vi "AOTF-Trigger_1.vi"(0 "Channel":string="1", 1 "Pulse length":i16[](array[numeric]), 2 "Sync trigger ratio":i32=20, 3 "error in (no error)":errorcluster caption="Fehler (Eingang, kein Fehler)", 4 "Triggered":bool, 5 "lp":dbl, 6 "ap":dbl) -> (7 "error out":errorcluster caption="Fehler (Ausgang)")   [LabVIEW 2011]
doc: "I. Description:\nThis example demonstrates how to generate a continuous digital pulse train from a Counter Output Channel started by an external digital trigger. The Frequency, Duty Cycle, and Idle State are all configurable. \n\nThis example shows how to configure the pulse in terms of Frequency/Duty Cycle, but can easily be modified to generate a pulse in terms of Time or Ticks.\n\nII. Instructions for Running:\n1. Select the Physical Channel which corresponds to the counter you want to output your signal to on the DAQ device.\n2. Enter the Frequency and Duty Cycle to define the pulse parameters. You can also change the Idle State to set the state the line will remain in after the generation is stopped. Additionally, you can set the Initial Delay (in seconds) which will delay the beginning of the pulse train from the start call; this is currently wired to 0.0 on the block diagram. \n3. Setup the Trigger Parameters. In this example the VI is expecting a Rising Edge Digital Trigger on PFI9. \n\nIII. Block Diagram Steps:\n1. Create a Counter Output channel to produce a Pulse in terms of Frequency. If the Idle State of the pulse is set to low the first transition of the generated signal is from low to high.\n2. Use the DAQmx Trigger VI to configure a trigger to start on a digital edge.\n2. Use the DAQmx Timing VI (Implicit) to configure the duration of the pulse generation.\n3. Call the Start VI to arm the counter and begin the pulse train generation.\n4. Loop continuously until the user presses the Stop button. Check for errors every 100 ms using the Is Task Done? VI\n5. Call the Clear Task VI to clear the Task.\n\nIV. I/O Connections Overview:\nThe counter will output the pulse train on the output terminal of the counter specified in the Physical Channel I/O control. \n\nIn this example the output will be sent to the default output terminal on ctr0.\n\nFor more information on the default counter input and output terminals for your device, open the NI-DAQmx Help, and refer to Counter Signal Connections found under the Device Considerations book in the table of contents."
uses:
  <vilib>/DAQmx/configure/timing.llb/DAQmx Timing (Implicit).vi
  <vilib>/Utility/error.llb/DialogType.ctl
  <vilib>/DAQmx/configure/trigger.llb/DAQmx Start Trigger (Digital Edge).vi
  <vilib>/DAQmx/write.llb/DAQmx Write (Digital Bool 1Line 1Point).vi
  <vilib>/DAQmx/read.llb/DAQmx Read (Digital Bool 1Line 1Point).vi
  <vilib>/DAQmx/create/channels.llb/DAQmx Create Channel (DI-Digital Input).vi
  <vilib>/DAQmx/create/channels.llb/DAQmx Create Channel (DO-Digital Output).vi
  <vilib>/DAQmx/create/channels.llb/DAQmx Create Channel (CO-Pulse Generation-Ticks).vi
  <vilib>/DAQmx/create/channels.llb/DAQmx Create Channel (CO-Pulse Generation-Frequency).vi
  <vilib>/DAQmx/create/channels.llb/DAQmx Create Channel (CO-Pulse Generation-Time).vi
panel:
  out "Delay":dbl[](array[numeric])
  out "Duty cycle":dbl[](array[numeric])
  # "Channel Parameters"
  # "Trigger Parameters"
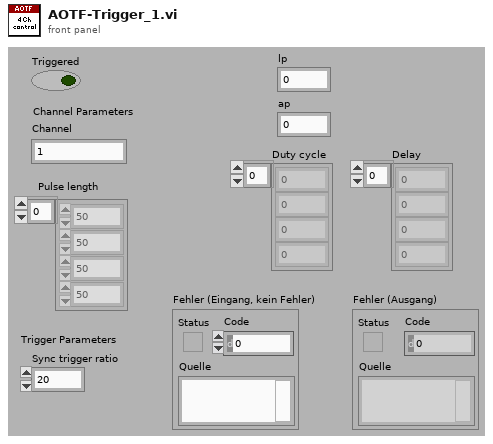
[diagram p1: front panel]
types:
  T1 = typedef "DialogType.ctl" = u16
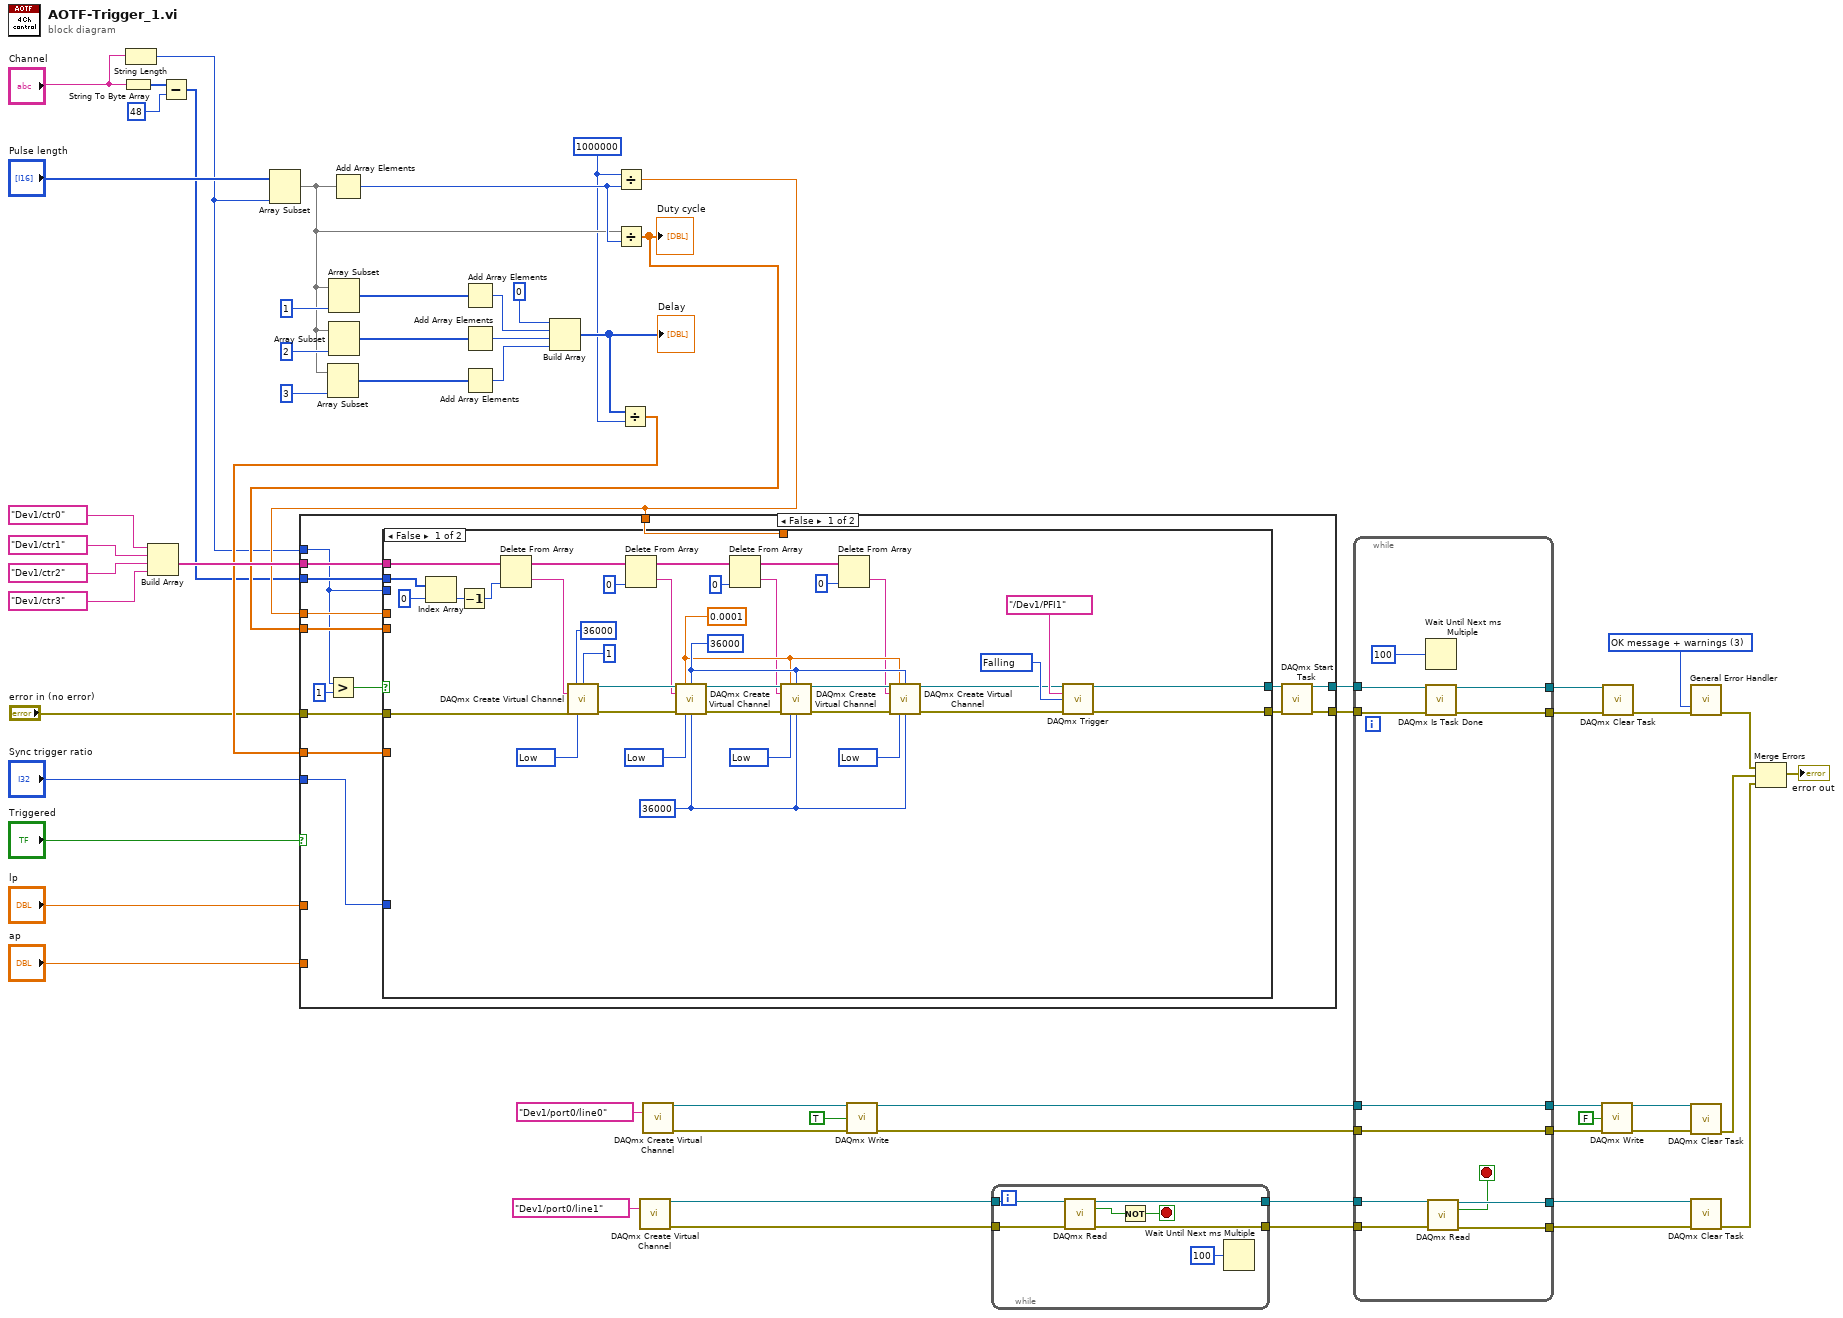
[diagram p0: block diagram]
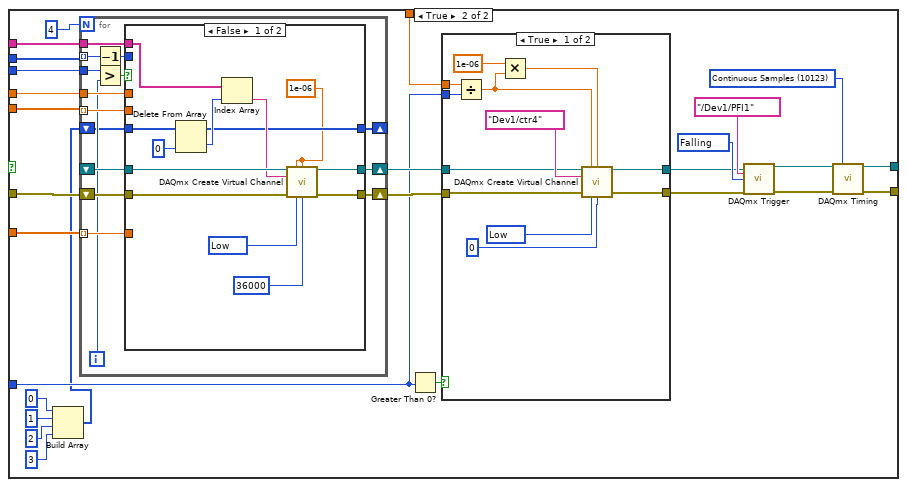
[diagram p2: hidden frame]
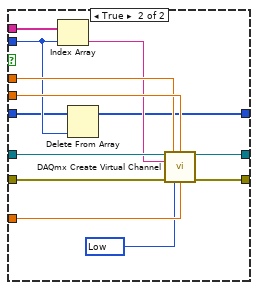
[diagram p4: hidden frame]
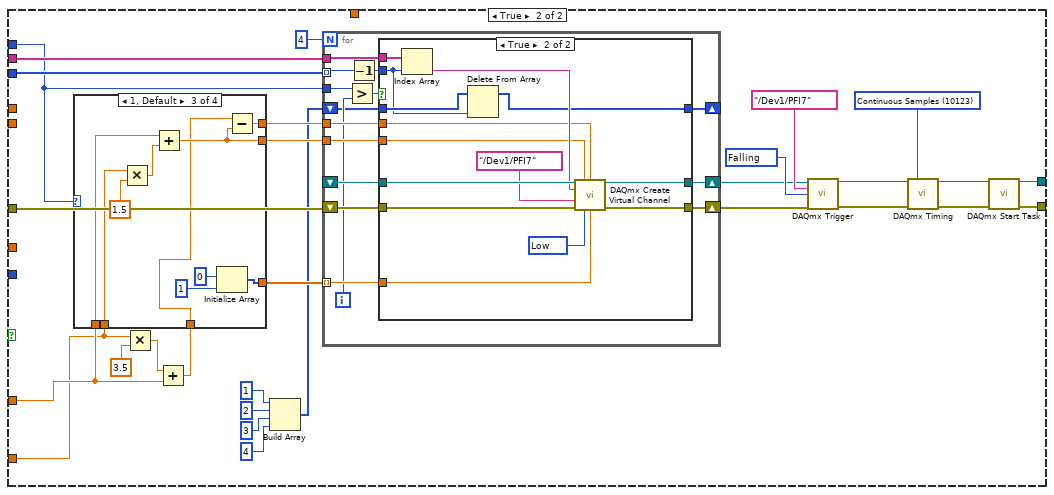
[diagram p5: hidden frame]
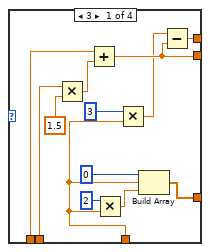
[diagram p6: hidden frame]
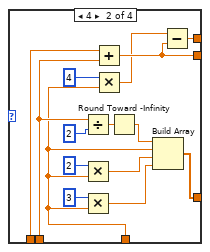
[diagram p7: hidden frame]
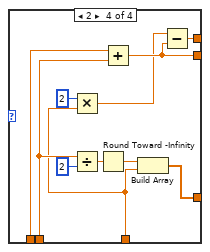
[diagram p8: hidden frame]
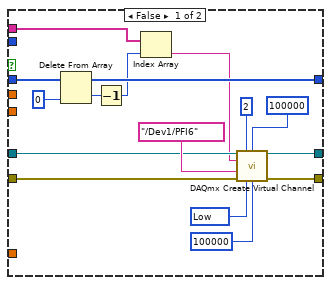
[diagram p9: hidden frame]
diagram:
  w38 = T1 3 items=["no dialog", "OK message", "continue or stop message", "OK message + warnings", "continue/stop + warnings"] ("type of dialog (OK msg:1)")
  w40 = 1000000
  n1 = String To Byte Array(string="Channel") -> (unsigned byte array=w60:u8[])
  n2 = String Length(string="Channel") -> (length=w2:i32)
  n3 = Build Array(tag "Dev1/ctr0" ("Counter 2"), tag "Dev1/ctr1" ("Counter 2"), tag "Dev1/ctr2" ("Counter 2"), tag "Dev1/ctr3" ("Counter 2")) -> (w15:tag[])
  n4 = Subtract(x=w60, y=48) -> (x-y=w1:i32[])
  n5 = Array Subset(array="Pulse length", length=w2) -> (w42:i16[])  [unwired: 1 in]
  n6 = Array Subset(array=w42, length=3) -> (w52:i16[])  [unwired: 1 in]
  n7 = Array Subset(array=w42, length=1) -> (w51:i16[])  [unwired: 1 in]
  n8 = Array Subset(array=w42, length=2) -> (w53:i16[])  [unwired: 1 in]
  n9 = Add Array Elements(numeric array=w42) -> (sum=w43:i16)
  n10 = Add Array Elements(numeric array=w51) -> (sum=w48:i16)
  n11 = Add Array Elements(numeric array=w53) -> (sum=w50:i16)
  n12 = Add Array Elements(numeric array=w52) -> (sum=w49:i16)
  n13 = Build Array(0, w48, w50, w49) -> (w41:i32[])
  "Delay" <- w41
  n14 = Divide(x=w40, y=w43) -> (x/y=w11:dbl)
  n15 = Divide(x=w42, y=w43) -> (x/y=w13:dbl[])
  "Duty cycle" <- w13
  n16 = Divide(x=w41, y=w40) -> (x/y=w14:dbl[])
  n17 = case shown="False" "Triggered" {
    tunnel: [w74 w224] -> w35
    tunnel: [w73 w223] -> w34
    tunnel: w15 -> [w71 w205]
    tunnel: w1 -> [w67 w215]
    tunnel: w14 -> [w70 _]
    tunnel: w13 -> [w68 _]
    tunnel: w11 -> [w69 _]
    tunnel: w2 -> [w63 w201]
    tunnel: "Sync trigger ratio" -> [w72 _]
    tunnel: w11 -> [w66 _]
    tunnel: "error in (no error)" -> [w65 w214]
    tunnel: "ap" -> [_ w208]
    tunnel: "lp" -> [_ w209]
    frame False {
      n18 = Greater?(x=w63, y=1) -> (0:w64:bool)
      n19 = case shown="False" w64 {
        tunnel: [w108 w140] -> w76
        tunnel: [w109 w139] -> w75
        tunnel: w72 -> [_ w130]
        tunnel: w71 -> [w111 w127]
        tunnel: w70 -> [_ w126]
        tunnel: w69 -> [_ w125]
        tunnel: w68 -> [_ w124]
        tunnel: w67 -> [w103 w123]
        tunnel: w63 -> [_ w116]
        tunnel: w66 -> [_ w122]
        tunnel: w65 -> [w110 w121]
        frame False {
          w88 = 36000
          w97 = 10214 items=["High"=10192, "Low"=10214] ("Idle State 2")
          w98 = 10214 items=["High"=10192, "Low"=10214] ("Idle State 2")
          w99 = 10214 items=["High"=10192, "Low"=10214] ("Idle State 2")
          w87 = 36000
          w86 = 0.0001
          w104 = 10214 items=["High"=10192, "Low"=10214] ("Idle State 2")
          w112 = u16 10171 items=["Falling"=10171, "Rising"=10280]
          n20 = Index Array(array=w103, index=0) -> (element=w101:i32)
          n21 = Decrement(x=w101) -> (x-1=w100:i32)
          n22 = Delete From Array(array=w111, index=w100) -> (deleted portion=w107:tag, array with subset deleted=w85:tag[])  [unwired: 1 in]
          n23 = call-poly <vilib>:"DAQmx Create Virtual Channel.vi"("high time"=36000, "low time"=1, "counter"=w107, "error in"=w110, "idle state"=w104) -> ("task out"=w89:refnum<k21>, "error out"=w96:errorcluster)  [unwired: 9 in]
          n24 = Delete From Array(array=w85, index=0) -> (deleted portion=w81:tag, array with subset deleted=w84:tag[])  [unwired: 1 in]
          n25 = call-poly <vilib>:"DAQmx Create Virtual Channel.vi"("task in"=w89, "high time"=w86, "low time"=w87, "counter"=w81, "error in"=w96, "idle state"=w99, "initial delay"=w88) -> ("task out"=w90:refnum<k21>, "error out"=w95:errorcluster)  [unwired: 7 in]
          n26 = Delete From Array(array=w84, index=0) -> (deleted portion=w80:tag, array with subset deleted=w83:tag[])  [unwired: 1 in]
          n27 = call-poly <vilib>:"DAQmx Create Virtual Channel.vi"("task in"=w90, "high time"=w86, "low time"=w87, "counter"=w80, "error in"=w95, "idle state"=w98, "initial delay"=w88) -> ("task out"=w91:refnum<k21>, "error out"=w94:errorcluster)  [unwired: 7 in]
          n28 = Delete From Array(array=w83, index=0) -> (deleted portion=w82:tag)  [unwired: 1 in, 1 out]
          n29 = call-poly <vilib>:"DAQmx Create Virtual Channel.vi"("task in"=w91, "high time"=w86, "low time"=w87, "counter"=w82, "error in"=w94, "idle state"=w97, "initial delay"=w88) -> ("task out"=w92:refnum<k21>, "error out"=w93:errorcluster)  [unwired: 7 in]
          n30 = call-poly <vilib>:"DAQmx Trigger.vi"("task/channels in"=w92, "source"=tag "/Dev1/PFI1" ("Trigger Source"), "edge"=w112, "error in"=w93) -> ("task out"=w109:refnum<k21>, "error out"=w108:errorcluster)  [unwired: 10 in]
        }
        frame True {
          w136 = u16 10171 items=["Falling"=10171, "Rising"=10280]
          w138 = 10123 items=["Finite Samples"=10178, "Continuous Samples"=10123] ("sample mode")
          n31 = Build Array(0, 1, 2, 3) -> (w114:i32[])
          n32 = for {
            N: 4 -> [_]
            shift-right: [w169] -> w132
            shift-left: w121 -> [w168]
            shift-right: [w167] -> w131
            shift-left: _ -> [w166]
            tunnel: w124 -> [w165] mode=indexing
            tunnel: w125 -> [w164]
            tunnel: w126 -> [w163] mode=indexing
            tunnel: w127 -> [w162]
            tunnel: w123 -> [w161] mode=indexing
            tunnel: w116 -> [w158]
            shift-right: [w155] -> _
            shift-left: w114 -> [w156]
            i -> [w159]
            n33 = Decrement(x=w161) -> (x-1=w157:i32)
            n34 = Greater?(x=w158, y=w159) -> (0:w160:bool)
            n35 = case shown="False" w160 {
              tunnel: [w181 w195] -> w169
              tunnel: w168 -> [w180 w194]
              tunnel: [w178 w193] -> w167
              tunnel: w166 -> [w179 w192]
              tunnel: w165 -> [_ w191]
              tunnel: w164 -> [_ w190]
              tunnel: w163 -> [_ w189]
              tunnel: w162 -> [w174 w187]
              tunnel: w157 -> [_ w185]
              tunnel: w156 -> [w176 w184]
              tunnel: [w172 w183] -> w155
              frame False {
                w170 = 1e-06
                w182 = 10214 items=["High"=10192, "Low"=10214] ("Idle State 2")
                n36 = Delete From Array(array=w176, index=0) -> (deleted portion=w175:i32, array with subset deleted=w172:i32[])  [unwired: 1 in]
                n37 = Index Array(array=w174, index=w175) -> (element=w173:tag)
                n38 = call-poly <vilib>:"DAQmx Create Virtual Channel.vi"("task in"=w179, "frequency"=w170, "duty cycle"=w170, "counter"=w173, "error in"=w180, "idle state"=w182, "initial delay"=36000) -> ("task out"=w178:refnum<k21>, "error out"=w181:errorcluster)  [unwired: 7 in]
              }
              frame True {
                w186 = 10214 items=["High"=10192, "Low"=10214] ("Idle State 2")
                n39 = Index Array(array=w187, index=w185) -> (element=w188:tag)
                n40 = Delete From Array(array=w184, index=w185) -> (array with subset deleted=w183:i32[])  [unwired: 1 in, 1 out]
                n41 = call-poly <vilib>:"DAQmx Create Virtual Channel.vi"("task in"=w192, "frequency"=w190, "duty cycle"=w191, "counter"=w188, "error in"=w194, "idle state"=w186, "initial delay"=w189) -> ("task out"=w193:refnum<k21>, "error out"=w195:errorcluster)  [unwired: 7 in]
              }
            }
          }
          n42 = Greater Than 0?(x=w130) -> (x > 0?=w133:bool)
          n43 = case shown="True" w133 {
            tunnel: [w151 w154] -> w128
            tunnel: [w148 w153] -> w129
            tunnel: w122 -> [w147 _]
            tunnel: w130 -> [w146 _]
            tunnel: w132 -> [w142 w153]
            tunnel: w131 -> [w141 w154]
            frame True {
              w149 = 10214 items=["High"=10192, "Low"=10214] ("Idle State 2")
              n44 = Divide(x=w147, y=w146) -> (x/y=w143:dbl)
              n45 = Multiply(x=1e-06, y=w143) -> (x*y=w145:dbl)
              n46 = call-poly <vilib>:"DAQmx Create Virtual Channel.vi"("task in"=w141, "frequency"=w143, "duty cycle"=w145, "counter"=tag "Dev1/ctr4" ("Counter 2"), "error in"=w142, "idle state"=w149, "initial delay"=0) -> ("task out"=w151:refnum<k21>, "error out"=w148:errorcluster)  [unwired: 7 in]
            }
            frame False {
            }
          }
          n47 = call-poly <vilib>:"DAQmx Trigger.vi"("task/channels in"=w128, "source"=tag "/Dev1/PFI1" ("Trigger Source"), "edge"=w136, "error in"=w129) -> ("task out"=w134:refnum<k21>, "error out"=w135:errorcluster)  [unwired: 10 in]
          n48 = call-poly <vilib>:"DAQmx Timing.vi"("task/channels in"=w134, "sample mode"=w138, "error in"=w135) -> ("task out"=w139:refnum<k21>, "error out"=w140:errorcluster)  [unwired: 11 in]
        }
      }
      n49 = call <vilib>:"DAQmx Start Task.vi"("task/channels in"=w75, "error in"=w76) -> ("task out"=w73:refnum<k21>, "error out"=w74:errorcluster)  [unwired: 12 in]
    }
    frame True {
      w220 = u16 10171 items=["Falling"=10171, "Rising"=10280]
      w222 = 10123 items=["Finite Samples"=10178, "Continuous Samples"=10123] ("sample mode")
      n50 = Multiply(x=w208, y=3.5) -> (x*y=w210:dbl)
      n51 = Add(x=w210, y=w209) -> (x+y=w207:dbl)
      n52 = case shown="1, Default" w201 {
        tunnel: w208 -> [w233 w248 w261 w268]
        tunnel: [w229 w244 w254 w267] -> w206
        tunnel: [w234 w247 w257 w270] -> w213
        tunnel: [w235 w250 w258 w271] -> w212
        tunnel: w209 -> [w232 w249 w262 w269]
        tunnel: w207 -> [w226 w238 w253 w264]
        frame 3 {
          n53 = Multiply(x=w233, y=1.5) -> (x*y=w236:dbl)
          n54 = Add(x=w232, y=w236) -> (x+y=w234:dbl)
          n55 = Multiply(x=2, y=w226) -> (x*y=w227:dbl)
          n56 = Multiply(x=3, y=w226) -> (x*y=w230:dbl)
          n57 = Build Array(0, w226, w227) -> (w229:dbl[])
          n58 = Subtract(x=w230, y=w234) -> (x-y=w235:dbl)
        }
        frame 4 {
          n59 = Divide(x=w248, y=2) -> (x/y=w251:dbl)
          n60 = Multiply(x=2, y=w238) -> (x*y=w241:dbl)
          n61 = Multiply(x=3, y=w238) -> (x*y=w240:dbl)
          n62 = Add(x=w249, y=w248) -> (x+y=w247:dbl)
          n63 = Multiply(x=4, y=w238) -> (x*y=w245:dbl)
          n64 = Round Toward -Infinity(1:w251) -> (0:w243:dbl)
          n65 = Build Array(w243, w238, w241, w240) -> (w244:dbl[])
          n66 = Subtract(x=w245, y=w247) -> (x-y=w250:dbl)
        }
        frame 1, Default {
          n67 = Multiply(x=w261, y=1.5) -> (x*y=w259:dbl)
          n68 = Add(x=w262, y=w259) -> (x+y=w257:dbl)
          n69 = Initialize Array(0, 1) -> (w254:i32[])
          n70 = Subtract(x=w253, y=w257) -> (x-y=w258:dbl)
        }
        frame 2 {
          n71 = Multiply(x=2, y=w264) -> (x*y=w265:dbl)
          n72 = Divide(x=w268, y=2) -> (x/y=w272:dbl)
          n73 = Round Toward -Infinity(1:w272) -> (0:w266:dbl)
          n74 = Add(x=w269, y=w268) -> (x+y=w270:dbl)
          n75 = Build Array(w266, w264) -> (w267:dbl[])
          n76 = Subtract(x=w265, y=w270) -> (x-y=w271:dbl)
        }
      }
      n77 = Build Array(1, 2, 3, 4) -> (w196:i32[])
      n78 = for {
        N: 4 -> [_]
        shift-right: [w288] -> w203
        shift-left: w214 -> [w287]
        shift-right: [w286] -> w204
        shift-left: _ -> [w285]
        tunnel: w205 -> [w283]
        tunnel: w215 -> [w276] mode=indexing
        tunnel: w206 -> [w282] mode=indexing
        tunnel: w213 -> [w281]
        tunnel: w212 -> [w280]
        tunnel: w201 -> [w277]
        shift-right: [w274] -> _
        shift-left: w196 -> [w275]
        i -> [w278]
        n79 = Greater?(x=w277, y=w278) -> (0:w279:bool)
        n80 = Decrement(x=w276) -> (x-1=w284:i32)
        n81 = case shown="True" w279 {
          tunnel: [w301 w318] -> w288
          tunnel: w287 -> [w302 w317]
          tunnel: [w299 w316] -> w286
          tunnel: w285 -> [w300 w315]
          tunnel: w284 -> [_ w306]
          tunnel: w283 -> [w295 w311]
          tunnel: w282 -> [_ w310]
          tunnel: w281 -> [_ w309]
          tunnel: w280 -> [_ w308]
          tunnel: w275 -> [w298 w307]
          tunnel: [w296 w305] -> w274
          frame False {
            w303 = 10214 items=["High"=10192, "Low"=10214] ("Idle State 2")
            n82 = Delete From Array(array=w298, index=0) -> (deleted portion=w294:i32, array with subset deleted=w296:i32[])  [unwired: 1 in]
            n83 = Decrement(x=w294) -> (x-1=w293:i32)
            n84 = Index Array(array=w295, index=w293) -> (element=w292:tag)
            n85 = call-poly <vilib>:"DAQmx Create Virtual Channel.vi"("task in"=w300, "high ticks"=2, "low ticks"=100000, "counter"=w292, "source of ticks"=tag "/Dev1/PFI6" ("Trigger Source"), "error in"=w302, "idle state"=w303, "initial delay"=100000) -> ("task out"=w299:refnum<k21>, "error out"=w301:errorcluster)  [unwired: 6 in]
          }
          frame True {
            w312 = 10214 items=["High"=10192, "Low"=10214] ("Idle State 2")
            n86 = Index Array(array=w311, index=w306) -> (element=w314:tag)
            n87 = Delete From Array(array=w307, index=w306) -> (array with subset deleted=w305:i32[])  [unwired: 1 in, 1 out]
            n88 = call-poly <vilib>:"DAQmx Create Virtual Channel.vi"("task in"=w315, "high ticks"=w309, "low ticks"=w308, "counter"=w314, "source of ticks"=tag "/Dev1/PFI7" ("Trigger Source"), "error in"=w317, "idle state"=w312, "initial delay"=w310) -> ("task out"=w316:refnum<k21>, "error out"=w318:errorcluster)  [unwired: 6 in]
          }
        }
      }
      n89 = call-poly <vilib>:"DAQmx Trigger.vi"("task/channels in"=w204, "source"=tag "/Dev1/PFI7" ("Trigger Source"), "edge"=w220, "error in"=w203) -> ("task out"=w217:refnum<k21>, "error out"=w216:errorcluster)  [unwired: 10 in]
      n90 = call-poly <vilib>:"DAQmx Timing.vi"("task/channels in"=w217, "sample mode"=w222, "error in"=w216) -> ("task out"=w219:refnum<k21>, "error out"=w218:errorcluster)  [unwired: 11 in]
      n91 = call <vilib>:"DAQmx Start Task.vi"("task/channels in"=w219, "error in"=w218) -> ("task out"=w223:refnum<k21>, "error out"=w224:errorcluster)  [unwired: 12 in]
    }
  }
  n92 = call-poly <vilib>:"DAQmx Create Virtual Channel.vi"("lines"=tag "Dev1/port0/line1" ("Counter 2")) -> ("task out"=w21:refnum<k21>, "error out"=w20:errorcluster)  [unwired: 13 in]
  n93 = call-poly <vilib>:"DAQmx Create Virtual Channel.vi"("lines"=tag "Dev1/port0/line0" ("Counter 2")) -> ("task out"=w16:refnum<k21>, "error out"=w17:errorcluster)  [unwired: 13 in]
  n94 = call-poly <vilib>:"DAQmx Write.vi"("task/channels in"=w16, "data"=TRUE, "error in"=w17) -> ("task out"=w24:refnum<k21>, "error out"=w25:errorcluster)  [unwired: 10 in, 1 out]
  n95 = while {
    tunnel: w21 -> [w325]
    tunnel: w20 -> [w324]
    tunnel: [w323] -> w19
    tunnel: [w322] -> w18
    stop <- w319 stop-if-true
    n96 = call-poly <vilib>:"DAQmx Read.vi"("task/channels in"=w325, "error in"=w324) -> ("task out"=w322:refnum<k21>, "data"=w320:bool, "error out"=w323:errorcluster)  [unwired: 11 in]
    n97 = Not(x=w320) -> (.not. x?=w319:bool)
    n98 = Wait Until Next ms Multiple(millisecond multiple=u32 100) -> ()  [unwired: 1 out]
  }
  n99 = while {
    tunnel: w35 -> [w336]
    tunnel: w34 -> [w337]
    tunnel: [w335] -> w36
    tunnel: [w334] -> w37
    tunnel: w18 -> [w330]
    tunnel: w19 -> [w329]
    tunnel: [w326] -> w29
    tunnel: [w327] -> w28
    tunnel: w24 -> [w327]
    tunnel: w25 -> [w326]
    tunnel: [w332] -> w22
    tunnel: [w331] -> w23
    stop <- w328 stop-if-true
    n100 = Wait Until Next ms Multiple(millisecond multiple=u32 100) -> ()  [unwired: 1 out]
    n101 = call <vilib>:"DAQmx Is Task Done.vi"("task/channels in"=w337, "error in"=w336) -> ("task out"=w335:refnum<k21>, "error out"=w334:errorcluster)  [unwired: 11 in, 1 out]
    n102 = call-poly <vilib>:"DAQmx Read.vi"("task/channels in"=w330, "error in"=w329) -> ("task out"=w331:refnum<k21>, "data"=w328:bool, "error out"=w332:errorcluster)  [unwired: 11 in]
  }
  n103 = call-poly <vilib>:"DAQmx Write.vi"("task/channels in"=w28, "data"=FALSE, "error in"=w29) -> ("task out"=w31:refnum<k21>, "error out"=w30:errorcluster)  [unwired: 10 in, 1 out]
  n104 = call <vilib>:"DAQmx Clear Task.vi"("task in"=w36, "error in"=w37) -> ("error out"=w61:errorcluster)  [unwired: 13 in]
  n105 = call <vilib>:"General Error Handler.vi"("type of dialog (OK msg:1)"=w38, "error in (no error)"=w61) -> ("error out"=w10:errorcluster)  [unwired: 9 in, 4 out]
  n106 = call <vilib>:"DAQmx Clear Task.vi"("task in"=w31, "error in"=w30) -> ("error out"=w9:errorcluster)  [unwired: 13 in]
  n107 = call <vilib>:"DAQmx Clear Task.vi"("task in"=w23, "error in"=w22) -> ("error out"=w8:errorcluster)  [unwired: 13 in]
  n108 = Merge Errors(w10, w9, w8) -> (→"error out":errorcluster)
